vi "formatCfgOutput.vi"(8 "error in (no error)":errorcluster, 10 "Log Message Queue":refnum<queue>, 11 "repoHandlers":refnum<class "repoHandler.lvclass">[](array[class])) -> (0 "error out":errorcluster, 2 "tableOutput":string[][](array[string]), 3 "repoHandlers":refnum<class "repoHandler.lvclass">[](array[class]))   [LabVIEW 2013]
uses:
  repoHandler/repoHandler.lvclass
  support/Message Queue/Message Cluster.ctl
  support/Message Queue/Enqueue Message (Single).vi
  support/Message Queue/repositoryConfigurator Message Queue.lvlib
panel:
  out "Numeric":i32
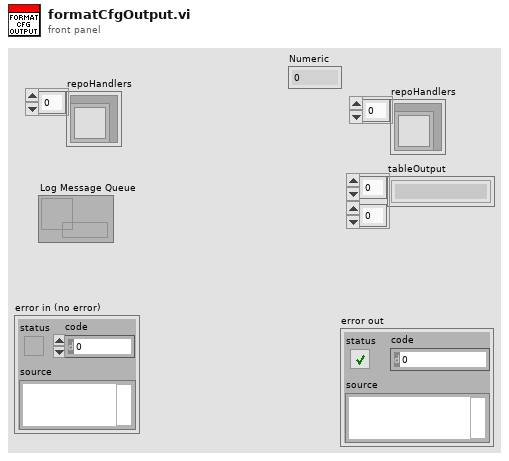
[diagram p1: front panel]
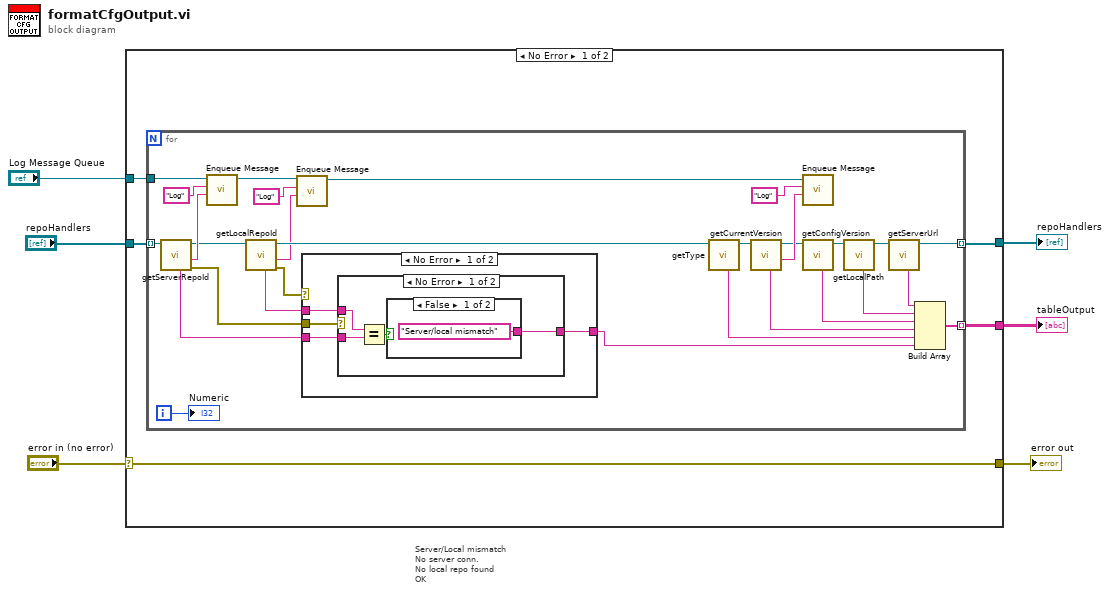
[diagram p0: block diagram]
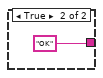
[diagram p2: hidden frame]
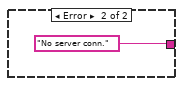
[diagram p3: hidden frame]
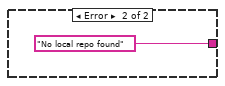
[diagram p4: hidden frame]
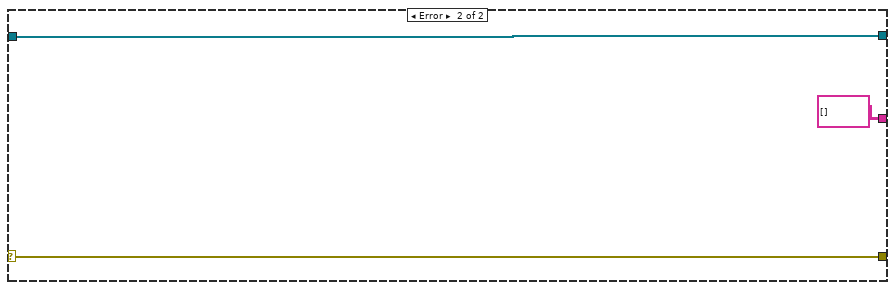
[diagram p5: hidden frame]
diagram:
  # "Server/Local mismatch\nNo server conn.\nNo local repo found\nOK"
  n1 = case shown="No Error" "error in (no error)" {
    selector: "error in (no error)" -> [w11 w55]
    tunnel: "repoHandlers" -> [w10 w53]
    tunnel: [w11 w55] -> w4
    tunnel: [w9 string[][] []] -> w3
    tunnel: "Log Message Queue" -> [w8 _]
    tunnel: [w7 w53] -> w1
    frame No Error {
      n2 = for {
        tunnel: w10 -> [w29] mode=indexing
        tunnel: [w40] -> w9 mode=indexing
        tunnel: w8 -> [w24]
        tunnel: [w12] -> w7 mode=indexing
        i -> [w35]
        n3 = call-dynamic "getServerRepoId.vi"("repoHandler in"=w29) -> ("error out"=w16:errorcluster, "Log"=w36:string, "repoHandler out"=w22:refnum<class "repoHandler.lvclass">, "ID"=w14:string)  [unwired: 7 in]
        n4 = call-poly "Enqueue Message.vi"("Message Data"=w36, "Message"="Log", "Message Queue"=w24) -> ("dup Message Queue"=w19:refnum<queue>)  [unwired: 7 in, 1 out]
        n5 = call-dynamic "getLocalRepoId.vi"("repoHandler in"=w22) -> ("error out"=w17:errorcluster, "Log"=w20:string, "repoHandler out"=w21:refnum<class "repoHandler.lvclass">, "ID"=w15:string)  [unwired: 7 in]
        n6 = call-poly "Enqueue Message.vi"("Message Data"=w20, "Message"="Log", "Message Queue"=w19) -> ("dup Message Queue"=w18:refnum<queue>)  [unwired: 7 in, 1 out]
        n7 = case shown="No Error" w17 {
          tunnel: w16 -> [w44 _]
          tunnel: w15 -> [w43 _]
          tunnel: w14 -> [w42 _]
          tunnel: [w41 "No local repo found"] -> w13
          frame No Error {
            n8 = case shown="No Error" w44 {
              tunnel: w43 -> [w48 _]
              tunnel: w42 -> [w47 _]
              tunnel: [w45 "No server conn." ("ID")] -> w41
              frame No Error {
                n9 = Equal?(x=w48, y=w47) -> (x = y?=w46:bool)
                n10 = case shown="False" w46 {
                  tunnel: ["Server/local mismatch" "OK"] -> w45
                  frame False {
                  }
                  frame True {
                  }
                }
              }
              frame Error {
              }
            }
          }
          frame Error {
          }
        }
        n11 = call-dynamic "getType.vi"("repoHandler in"=w21) -> ("repoHandler out"=w28:refnum<class "repoHandler.lvclass">, "Type"=w30:string)  [unwired: 8 in, 1 out]
        n12 = call-dynamic "getCurrentVersion.vi"("repoHandler in"=w28) -> ("Log"=w38:string, "repoHandler out"=w27:refnum<class "repoHandler.lvclass">, "Local Version"=w31:string)  [unwired: 7 in, 1 out]
        n13 = call-poly "Enqueue Message.vi"("Message Data"=w38, "Message"="Log", "Message Queue"=w18) -> ()  [unwired: 7 in, 2 out]
        n14 = call-dynamic "getConfigVersion.vi"("repoHandler in"=w27) -> ("repoHandler out"=w26:refnum<class "repoHandler.lvclass">, "Config Version"=w32:string)  [unwired: 8 in, 1 out]
        n15 = call-dynamic "getLocalPath.vi"("repoHandler in"=w26) -> ("repoHandler out"=w25:refnum<class "repoHandler.lvclass">, "Local Path"=w33:string)  [unwired: 8 in, 1 out]
        n16 = call-dynamic "getServerUrl.vi"("repoHandler in"=w25) -> ("repoHandler out"=w12:refnum<class "repoHandler.lvclass">, "Server url"=w34:string)  [unwired: 8 in, 1 out]
        n17 = Build Array(w34, w33, w32, w31, w30, w13) -> (w40:string[])
        "Numeric" <- w35
      }
    }
    frame Error {
    }
  }
  "error out" <- w4
  "tableOutput" <- w3
  "repoHandlers" <- w1
